vi "error.From JSON Tree.vi"(8 "error in (no error)":errorcluster, 10 "JSON Value in":variant, 11 "error in":refnum<class "error.lvclass">) -> (0 "error out":errorcluster, 3 "error out":refnum<class "error.lvclass">)   [LabVIEW 2020, in "JSON-RPC Lib.lvlib" / "error.lvclass"]
uses:
  error.lvclass
  error.lvclass/error.ctl
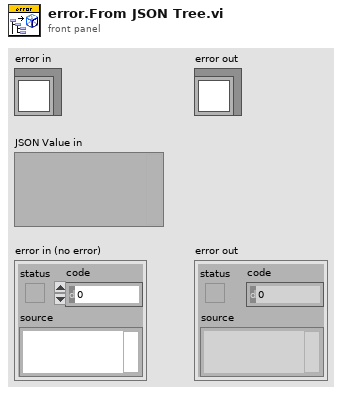
[diagram p1: front panel]
types:
  T1 = cluster{"code":i32, "message":string, "data":variant}
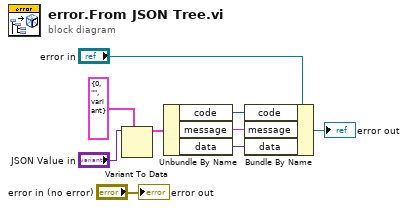
[diagram p0: block diagram]
diagram:
  n1 = Variant To Data(type=T1 {"code"=0, "message"="", "data"=variant} ("Cluster of class private data"), Variant="JSON Value in") -> (data=w4:T1)  [unwired: 1 in, 1 out]
  n2 = Unbundle By Name(w4) -> ("code"=w3:i32, "message"=w2:string, "data"=w1:variant)
  n3 = Bundle By Name(cluster="error in", "code"=w3, "message"=w2, "data"=w1) -> (→"error out":refnum<class "error.lvclass">)
  "error out" <- "error in (no error)"
